vi "Unflatten from String with Little-Endian Data.vi"() -> ()   [LabVIEW 2020]
doc: "This example takes a sample of binary data, parses the header information, and transforms it into an array of decimal points with the Unflatten from String function. This array is then plotted onto a waveform graph. It is very common for instruments to return binary data in this format.\n\nThe header consists of 3 parts:\nIt starts with the '#' sign. Immediately following this is a single digit number that denotes the number of digits that represent the byte count of this binary data. After this digit is the byte count, in the specified number of digits. After the header is the binary data. This data can be displayed in 3 ways -- Normal (Ascii), '\\' codes, and Hex values.\n\nFor example, \"#42000\" means that this binary data header has 4 digits that represent the byte count, and the byte count itself is 2000 bytes. You can use this information to accurately extract the correct amount of binary data."
panel:
  out "Unflattened Data":i16[](graph)
  # "Overview: Demonstrates the use of the Unflatten from String function to convert binary data to a numeric array.\nInstructions:\nRun the VI. The sample binary data will be unflattened from 2-byte, little-endian binary format to a numeric array and displayed in the graph."
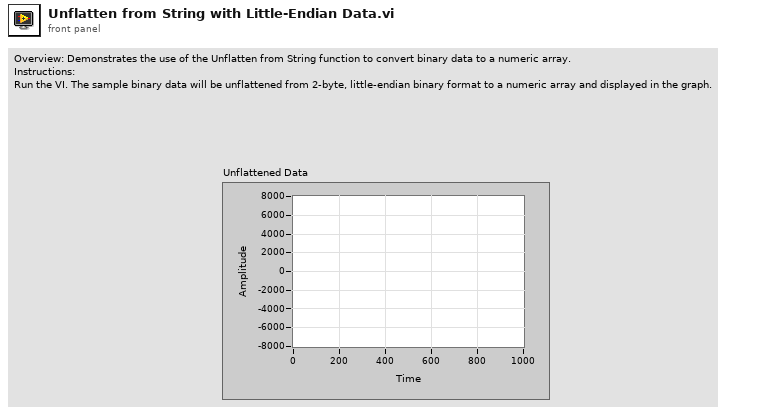
[diagram p1: front panel]
types:
  T1 = enum16{"big-endian, network order", "native, host order", "little-endian"}
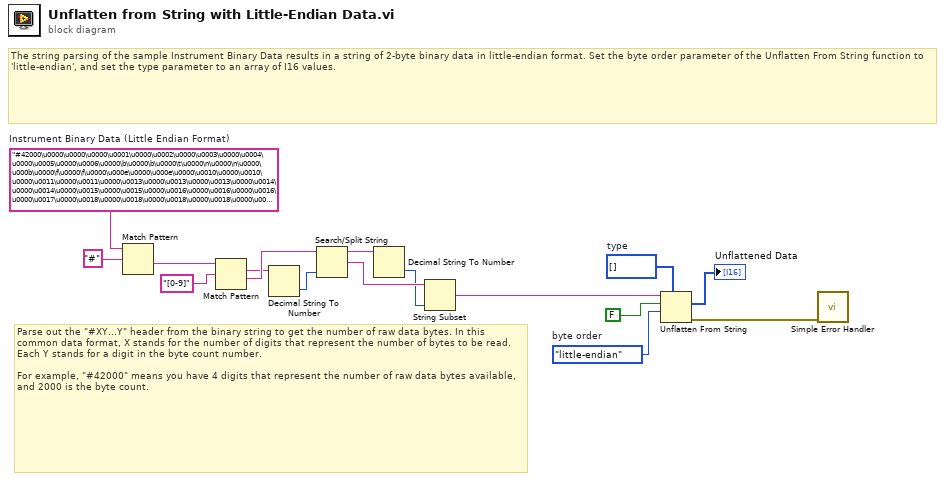
[diagram p0: block diagram]
diagram:
  w1 = "#42000\u0000\u0000\u0000\u0001\u0000\u0002\u0000\u0003\u0000\u0004\u0000\u0005\u0000\u0006\u0000\b\u0000\b\u0000\t\u0000\n\u0000\n\u0000\u000b\u0000\f\u0000\f\u0000\u000e\u0000\u000e\u0000\u0010\u0000\u0010\u0000\u0011\u0000\u0011\u0000\u0013\u0000\u0013\u0000\u0013\u0000\u0014\u0000\u0014\u0000\u0015\u0000\u0015\u0000\u0016\u0000\u0016\u0000\u0016\u0000\u0017\u0000\u0018\u0000\u0018\u0000\u0018\u0000\u0018\u0000\u0018\u0000\u0018\u0000\u0019\u0000\u0019\u0000\u0018\u0000\u0018\u0000\u0019\u0000\u0019\u0000\u0019\u0000\u0019\u0000\u0018\u0000\u0018\u0000\u0018\u0000\u0017\u0000\u0017\u0000\u0017\u0000\u0017\u0000\u0017\u0000\u0016\u0000\u0015\u0000\u0015\u0000\u0015\u0000\u0014\u0000\u0014\u0000\u0013\u0000\u0012\u0000\u0012\u0000\u0011\u0000\u0010\u0000\u000f\u0000\u000f\u0000\u000e\u0000\r\u0000\f\u0000\u000b\u0000\u000b\u0000\n\u0000\b\u0000\b\u0000\u0006\u0000\u0006\u0000\u0005\u0000\u0004\u0000\u0004\u0000\u0003\u0000\u0001\u0000\u0001\u0000\u0000\u0000ÿ\u0000þ\u0000ý\u0000ý\u0000û\u0000ù\u0000ú\u0000ø\u0000÷\u0000÷\u0000ö\u0000õ\u0000ô\u0000ò\u0000ò\u0000ñ\u0000ñ\u0000ð\u0000ï\u0000ï\u0000î\u0000í\u0000í\u0000ì\u0000ì\u0000ë\u0000ê\u0000ê\u0000ê\u0000é\u0000é\u0000è\u0000è\u0000è\u0000ç\u0000è\u0000ç\u0000ç\u0000ç\u0000ç\u0000ç\u0000ç\u0000ç\u0000ç\u0000è\u0000è\u0000è\u0000è\u0000ç\u0000è\u0000è\u0000é\u0000é\u0000ê\u0000ê\u0000ë\u0000ë\u0000ì\u0000ì\u0000í\u0000í\u0000î\u0000ï\u0000ï\u0000ð\u0000ð\u0000ñ\u0000ó\u0000ó\u0000ó\u0000ö\u0000ö\u0000ö\u0000ø\u0000ø\u0000ú\u0000ú\u0000û\u0000ü\u0000ý\u0000þ\u0000ÿ\u0000\u0000\u0000\u0001\u0000\u0001\u0000\u0002\u0000\u0003\u0000\u0004\u0000\u0005\u0000\u0006\u0000\u0007\u0000\b\u0000\b\u0000\n\u0000\u000b\u0000\f\u0000\r\u0000\r\u0000\u000e\u0000\u000e\u0000\u0010\u0000\u0010\u0000\u0011\u0000\u0011\u0000\u0013\u0000\u0013\u0000\u0014\u0000\u0014\u0000\u0015\u0000\u0015\u0000\u0016\u0000\u0016\u0000\u0017\u0000\u0017\u0000\u0017\u0000\u0018\u0000\u0018\u0000\u0019\u0000\u0018\u0000\u0019\u0000\u0019\u0000\u0019\u0000\u0019\u0000\u0019\u0000\u0019\u0000\u001a\u0000\u0019\u0000\u0019\u0000\u0019\u0000\u0018\u0000\u0019\u0000\u0018\u0000\u0018\u0000\u0018\u0000\u0017\u0000\u0017\u0000\u0017\u0000\u0015\u0000\u0015\u0000\u0015\u0000\u0014\u0000\u0013\u0000\u0014\u0000\u0013\u0000\u0012\u0000\u0012\u0000\u0011\u0000\u0010\u0000\u000f\u0000\u000f\u0000\u000e\u0000\r\u0000\f\u0000\u000b\u0000\u000b\u0000\n\u0000\t\u0000\b\u0000\u0007\u0000\u0006\u0000\u0005\u0000\u0004\u0000\u0002\u0000\u0002\u0000\u0001\u0000\u0000\u0000ÿ\u0000þ\u0000þ\u0000ü\u0000ü\u0000û\u0000ú\u0000ù\u0000ø\u0000÷\u0000÷\u0000õ\u0000õ\u0000ô\u0000ó\u0000ò\u0000ñ\u0000ð\u0000ï\u0000ï\u0000î\u0000î\u0000í\u0000ì\u0000ì\u0000ì\u0000ë\u0000ê\u0000ê\u0000ê\u0000é\u0000é\u0000é\u0000è\u0000è\u0000ç\u0000è\u0000è\u0000ç\u0000ç\u0000æ\u0000ç\u0000æ\u0000ç\u0000ç\u0000ç\u0000ç..."  # Instrument Binary Data (Little Endian Format)
  w12 = T1."little-endian"  # byte order
  w15 = i16[] []  # type
  # "Parse out the \"#XY...Y\" header from the binary string to get the number of raw data bytes. In this common data format, X stands for the number of digits that represent the number of bytes to be read. Each Y stands for a digit in the byte count number.\n\nFor example, \"#42000\" means you have 4 digits that represent the number of raw data bytes available, and 2000 is the byte count."
  # "The string parsing of the sample Instrument Binary Data results in a string of 2-byte binary data in little-endian format. Set the byte order parameter of the Unflatten From String function to 'little-endian', and set the type parameter to an array of I16 values."
  n1 = Match Pattern(string=w1, regular expression="#" ("format string")) -> (after substring=w6:string)  [unwired: 1 in, 3 out]
  n2 = Match Pattern(string=w6, regular expression="[0-9]") -> (match substring=w7:string, after substring=w8:string)  [unwired: 1 in, 2 out]
  n3 = Decimal String To Number(string=w7) -> (number=w11:i32)  [unwired: 3 out]
  n4 = Search/Split String(string=w8, offset (0)=w11) -> (substring before match=w9:string, match + rest of string=w10:string)  [unwired: 1 in, 1 out]
  n5 = Decimal String To Number(string=w9) -> (number=w4:i32)  [unwired: 3 out]
  n6 = String Subset(string=w10, length (rest)=w4) -> (substring=w3:string)  [unwired: 1 out]
  n7 = Unflatten From String(type=w15, binary string=w3, data includes array or string size? (T)=FALSE, byte order (0:big-endian, network order)=w12) -> (value=→"Unflattened Data":i16[], error out=w16:errorcluster)  [unwired: 1 in, 1 out]
  n8 = call <vilib>:"Simple Error Handler.vi"("error in (no error)"=w16) -> ()  [unwired: 4 in, 5 out]
